vi "ROS_subscriber.vi"() -> ()   [LabVIEW 2017]
uses:
  <vilib>/Tufts CEEO ROS for LabVIEW Software/ROS/Code/Console/Servers/ServerSubs/TopicDef.ctl
  <vilib>/Tufts CEEO ROS for LabVIEW Software/ROS/Code/SubVIs/_ROSDirection.ctl
  Simulator_SupportedVIs/Ctl/Current_Position.ctl
panel:
  out "Obs":cluster{i32[], i32[]}(graph)
  out "error out":errorcluster
  in  "stop":bool
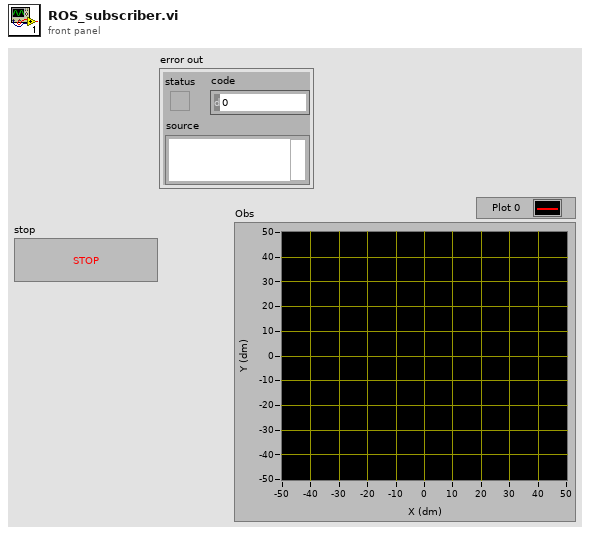
[diagram p1: front panel]
types:
  T1 = typedef "TopicDef.ctl" = cluster{"Topic":string, "Type":string, "Action":T2, "Update (ms)":u16, "queue size":u16}
  T2 = typedef "_ROSDirection.ctl" = enum16{"Node", "Publisher", "Subscriber", "ServiceClient", "ServiceProvider"}
  T3 = typedef "_ROSControl.ctl" = cluster{"topic port":u16, "Node":string, "topic":string, "type":string, "node port":u16, "error ":errorcluster, "Direction":T2, "Update (ms)":u16, "FIFO size":u16}
  T4 = typedef "Current_Position.ctl" = cluster{"X":dbl, "Y":dbl, "Theta":dbl}
  T5 = typedef "LaserScan.ctl" = cluster{"LaserScan_Header":cluster{"Seq":u32, "Frame ID":string, cluster{"Seconds":i32, "Nanoseconds":i32}}, "angle_min":dbl, "angle_max":dbl, "angle_increment":dbl, "time_increment":dbl, "scan_time":dbl, "range_min":dbl, "range_max":dbl, "ranges[]":dbl[], "intensities[]":dbl[]}
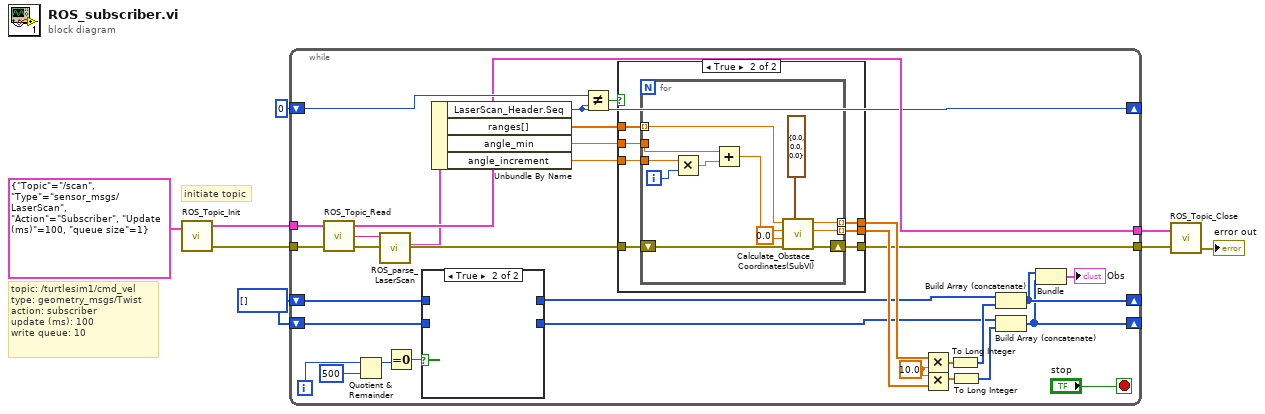
[diagram p0: block diagram]
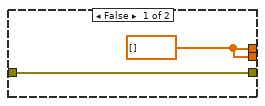
[diagram p3: hidden frame]
diagram:
  w6 = i32[] []
  # "initiate topic"
  # "topic: /turtlesim1/cmd_vel\ntype: geometry_msgs/Twist\naction: subscriber\nupdate (ms): 100\nwrite queue: 10"
  n1 = call <vilib>:"ROS_Topic_Init.vi"("Definitions"=T1 {"Topic"="/scan", "Type"="sensor_msgs/LaserScan", "Action"=enum."Subscriber", "Update (ms)"=100, "queue size"=1}) -> ("ROS out"=w3:T3, "error out"=w4:errorcluster)  [unwired: 2 in]
  n2 = while {
    shift-right: [w18] -> _
    shift-left: u32 0 ("Seq") -> [w40]
    shift-right: [w27] -> _
    shift-left: w6 -> [w12]
    shift-right: [w26] -> _
    shift-left: w6 -> [w11]
    tunnel: w4 -> [w24]
    tunnel: w3 -> [w23]
    tunnel: [w20] -> w2
    tunnel: [w19] -> w1
    i -> [w16]
    stop <- "stop" stop-if-true
    w35 = 10.0 ("y")
    n3 = call <vilib>:"ROS_Topic_Read.vi"("error in (no error)"=w24, "ROS in"=w23) -> ("error out"=w21:errorcluster, "Reply"=w22:string, "ROS out"=w19:T3)  [unwired: 1 in]
    n4 = Quotient & Remainder(x=w16, y=500) -> (x-y*floor(x/y)=w14:i32)  [unwired: 1 out]
    n5 = call "ROS_parse_LaserScan.vi"("msg in"=w22) -> ("LaserScan_msg"=w17:T5)  [unwired: 9 in, 1 out]
    n6 = Equal To 0?(x=w14) -> (x = 0?=w13:bool)
    n7 = case shown="True" w13 {
      tunnel: w12 -> [w42 _]
      tunnel: w11 -> [w41 _]
      tunnel: [w42 _] -> w10
      tunnel: [w41 _] -> w9
      frame False {
      }
      frame True {
      }
    }
    n8 = Unbundle By Name(w17) -> ("LaserScan_Header.Seq"=w18:u32, "ranges[]"=w37:dbl[], "angle_min"=w38:dbl, "angle_increment"=w36:dbl)
    n9 = Not Equal?(x=w40, y=w18) -> (x != y?=w39:bool)
    n10 = case shown="True" w39 {
      tunnel: w38 -> [_ w50]
      tunnel: w37 -> [_ w51]
      tunnel: w36 -> [_ w49]
      tunnel: [w44 w48] -> w30
      tunnel: [w44 w47] -> w29
      tunnel: w21 -> [w43 w46]
      tunnel: [w43 w45] -> w20
      frame False {
        w44 = dbl[] []
      }
      frame True {
        n11 = for {
          tunnel: w51 -> [w52] mode=indexing
          tunnel: w50 -> [w53]
          tunnel: w49 -> [w54]
          tunnel: [w58] -> w48 mode=indexing
          tunnel: [w57] -> w47 mode=indexing
          shift-right: [w55] -> w45
          shift-left: w46 -> [w56]
          i -> [w63]
          n12 = Multiply(x=w54, y=w63) -> (x*y=w62:dbl)
          n13 = Add(x=w53, y=w62) -> (x+y=w61:dbl)
          n14 = call "Calculate_Obstace_Coordinates(SubVI).vi"("Current_Position_in"=T4 {"X"=0.0, "Y"=0.0, "Theta"=0.0}, "error in (no error)"=w56, "SensorPos"=0.0 ("ServoPos"), "SensorAngle"=w61, "ObsDistance"=w52) -> ("error out"=w55:errorcluster, "Y_obs"=w57:dbl, "X_obs"=w58:dbl)  [unwired: 3 in, 1 out]
        }
      }
    }
    n15 = Multiply(x=w30, y=w35) -> (x*y=w34:dbl[])
    n16 = Multiply(x=w35, y=w29) -> (x*y=w33:dbl[])
    n17 = To Long Integer(number=w34) -> (32bit integer=w32:i32[])
    n18 = To Long Integer(number=w33) -> (32bit integer=w31:i32[])
    n19 = Build Array (concatenate)(w10, w32) -> (w27:i32[])
    n20 = Build Array (concatenate)(w9, w31) -> (w26:i32[])
    n21 = Bundle(w27, w26) -> (→"Obs":cluster{i32[], i32[]})  [unwired: 1 in]
  }
  n22 = call <vilib>:"ROS_Topic_Close.vi"("error in"=w2, "ROS in"=w1) -> ("error out"=→"error out":errorcluster)  [unwired: 2 in]
